vi "Perturb Current Solution.vi"(11 "Solution":T1) -> (3 "Schedule":u16[](array[numeric]))   [LabVIEW 2013, in "SA.lvclass"]
uses:
  SA.lvclass
  Controls/Solution_SA.ctl
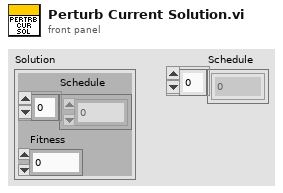
[diagram p1: front panel]
types:
  T1 = typedef "Solution_SA.ctl" = cluster{"Schedule":u16[], "Fitness":i16}
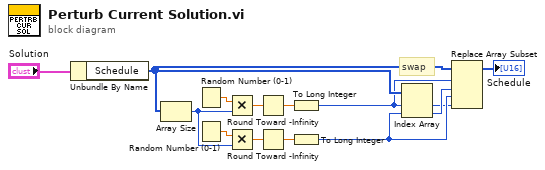
[diagram p0: block diagram]
diagram:
  # "swap"
  n1 = Unbundle By Name("Solution") -> ("Schedule"=w7:u16[])
  n2 = Array Size(array=w7) -> (size(s)=w10:i32)
  n3 = Random Number (0-1)() -> (number: 0 to 1=w12:dbl)
  n4 = Random Number (0-1)() -> (number: 0 to 1=w11:dbl)
  n5 = Multiply(x=w12, y=w10) -> (x*y=w9:dbl)
  n6 = Multiply(x=w11, y=w10) -> (x*y=w8:dbl)
  n7 = Round Toward -Infinity(1:w9) -> (0:w6:dbl)
  n8 = Round Toward -Infinity(1:w8) -> (0:w5:dbl)
  n9 = To Long Integer(number=w6) -> (32bit integer=w4:i32)
  n10 = To Long Integer(number=w5) -> (32bit integer=w2:i32)
  n11 = Index Array(array=w7, index #1=w4, index #2=w2) -> (element #1=w1:u16, element #2=w3:u16)
  n12 = Replace Array Subset(array=w7, new element #1=w3, index #1=w4, new element #2=w1, index #2=w2) -> (→"Schedule":u16[])
